vi "parse gentec acquire string.vi"(11 "Acquisition String":string) -> (2 "Channel 2 value":dbl, 3 "Channel 1 value":dbl)   [LabVIEW 2020, in "Gentec SlinkUSB.lvclass"]
uses:
  Gentec SlinkUSB.lvclass
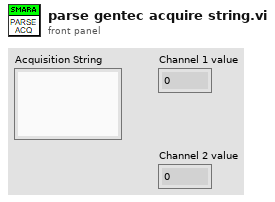
[diagram p1: front panel]
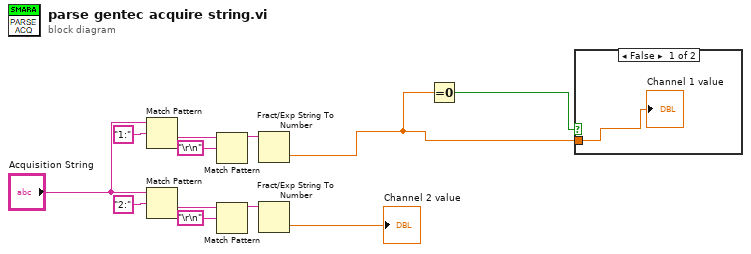
[diagram p0: block diagram]
diagram:
  n1 = Match Pattern(string="Acquisition String", regular expression="1:") -> (after substring=w7:string)  [unwired: 1 in, 3 out]
  n2 = Match Pattern(string="Acquisition String", regular expression="2:") -> (after substring=w11:string)  [unwired: 1 in, 3 out]
  n3 = Match Pattern(string=w7, regular expression="\r\n") -> (before substring=w8:string)  [unwired: 1 in, 3 out]
  n4 = Match Pattern(string=w11, regular expression="\r\n") -> (before substring=w12:string)  [unwired: 1 in, 3 out]
  n5 = Fract/Exp String To Number(string=w8) -> (number=w1:dbl)  [unwired: 3 in, 1 out]
  n6 = Fract/Exp String To Number(string=w12) -> (number=→"Channel 2 value":dbl)  [unwired: 3 in, 1 out]
  n7 = Equal To 0?(x=w1) -> (x = 0?=w2:bool)
  n8 = case shown="False" w2 {
    tunnel: w1 -> [w13 _]
    frame False {
      "Channel 1 value" <- w13
    }
    frame True {
    }
  }
